vi "Serial CAM Buffer Handler.vi"(7 "Serials buffer operations":T1(ring), 8 "error in (no error)":errorcluster, 10 "Status":string, 11 "Serial":string) -> (0 "error out":errorcluster, 2 "number of serials":i32, 3 "poped serial":string)   [LabVIEW 2024]
panel:
  out "Buffer":string[][](array[string])
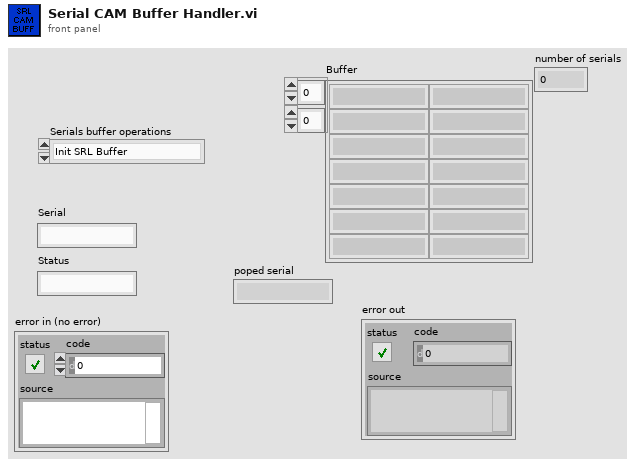
[diagram p1: front panel]
types:
  T1 = enum16{"Init SRL Buffer", "Insert SRL in Buffer", "Insert SRL Status", "Remove SRL from Buffer", "pop serial"}
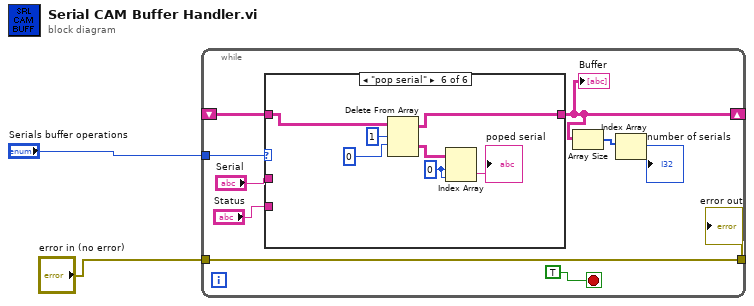
[diagram p0: block diagram]
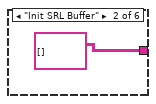
[diagram p3: hidden frame]
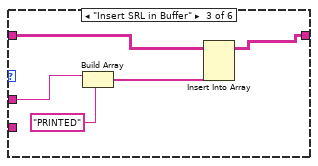
[diagram p4: hidden frame]
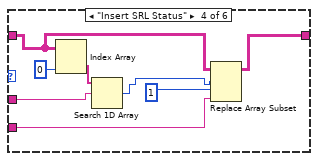
[diagram p5: hidden frame]
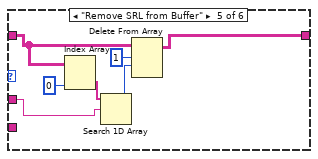
[diagram p6: hidden frame]
diagram:
  n1 = while {
    tunnel: "Serials buffer operations" -> [w11]
    shift-right: [w6] -> _
    shift-left: _ -> [w10]
    tunnel: [w7] -> w2
    tunnel: "error in (no error)" -> [w7]
    stop <- TRUE stop-if-true
    n2 = case shown="\"pop serial\"" w11 {
      tunnel: [w13 string[][] [] ("Buffer") w16 w20 w34 w41] -> w6
      tunnel: w10 -> [w13 _ w19 w24 w31 w40]
      tunnel: "Serial" -> [_ _ w15 w25 w30 _]
      tunnel: "Status" -> [_ _ _ w21 _ _]
      frame Default {
      }
      frame "Init SRL Buffer" {
      }
      frame "Insert SRL in Buffer" {
        n3 = Build Array(w15, "PRINTED" ("element")) -> (w17:string[])
        n4 = Insert Into Array(array=w19, new element=w17) -> (w16:string[][])  [unwired: 2 in]
      }
      frame "Insert SRL Status" {
        n5 = Index Array(array=w24, index (col)=0 ("disabled index (col)")) -> (element=w26:string[])  [unwired: 1 in]
        n6 = Search 1D Array(1D array=w26, element=w25) -> (index of element=w23:i32)  [unwired: 1 in]
        n7 = Replace Array Subset(array=w24, new element=w21, index (row)=w23, index (col)=1) -> (w20:string[][])
      }
      frame "Remove SRL from Buffer" {
        n8 = Index Array(array=w31, index (col)=0 ("disabled index (col)")) -> (element=w32:string[])  [unwired: 1 in]
        n9 = Search 1D Array(1D array=w32, element=w30) -> (index of element=w29:i32)  [unwired: 1 in]
        n10 = Delete From Array(array=w31, length=1, index (row)=w29) -> (array with subset deleted=w34:string[][])  [unwired: 1 in, 1 out]
      }
      frame "pop serial" {
        w36 = 0 ("index (row)")
        n11 = Delete From Array(array=w40, length=1, index (row)=0) -> (deleted portion=w37:string[][], array with subset deleted=w41:string[][])  [unwired: 1 in]
        n12 = Index Array(array=w37, index (row)=w36, index (col)=w36) -> (element=→"poped serial":string)
      }
    }
    "Buffer" <- w6
    n13 = Array Size(array=w6) -> (size(s)=w5:i32[])
    n14 = Index Array(array=w5) -> (element=→"number of serials":i32)  [unwired: 1 in]
  }
  "error out" <- w2
